vi "Unmap Shared Memory.vi"(8 "error in (no error)":errorcluster, 11 "shared memory in":T1) -> (0 "error out":errorcluster, 3 "shared memory out":T1)   [LabVIEW 2013, in "Linux RT IPC.lvlib" / "Shared Memory.lvlib" / "Shared Memory.lvclass"]
doc: "This performs the opposite operation of the Map Shared Memory VI, which is to unmap the shared memory from the calling process (LabVIEW). This invalidates the pointer previously returned by the Map VI."
uses:
  Shared Memory.lvclass
  Controls/reference.ctl
  Shared Memory.lvlib
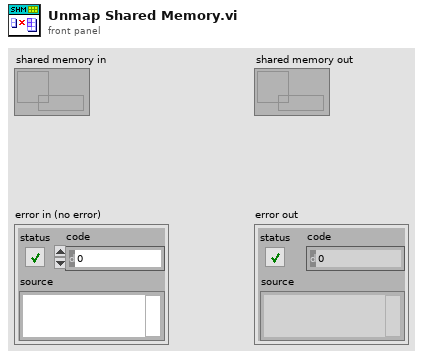
[diagram p1: front panel]
types:
  T1 = typedef "Linux RT IPC.lvlib/Shared Memory.lvlib/reference.ctl" = refnum<data-value>
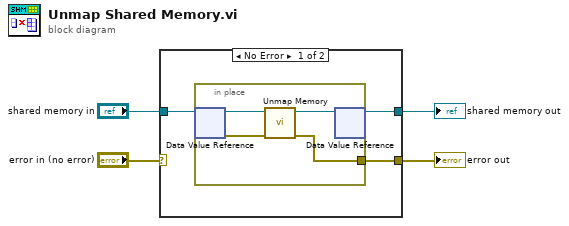
[diagram p0: block diagram]
diagram:
  n1 = case shown="No Error" "error in (no error)" {
    selector: "error in (no error)" -> [_ w13]
    tunnel: [w5 w13] -> w4
    tunnel: "shared memory in" -> [w7 w12]
    tunnel: [w6 w12] -> w1
    frame No Error {
      n2 = in-place {
        in-place-border: [w8] -> w5
        n3 = in-place-dvr #1(w7) -> (w11:refnum<class "Shared Memory.lvclass">, w10:errorcluster)
        n4 = call "Unmap Memory.vi"("error in (no error)"=w10, "Shared Memory in"=w11) -> ("error out"=w8:errorcluster, "Shared Memory out"=w9:refnum<class "Shared Memory.lvclass">)  [unwired: 8 in]
        n5 = in-place-dvr #1(w9) -> (w6:T1)  [unwired: 1 out]
      }
    }
    frame Error {
    }
  }
  "error out" <- w4
  "shared memory out" <- w1
